vi "integration_code_python.vi"(1 "path de l'image":string, 2 "IDs acceptés":dbl[](array[numeric])) -> (0 "validation":bool)   [LabVIEW 2020]
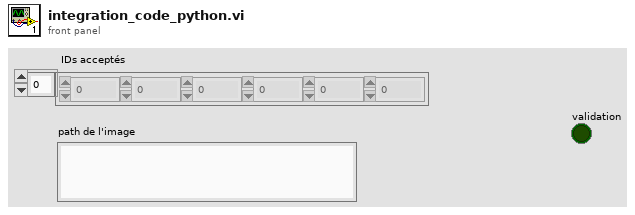
[diagram p1: front panel]
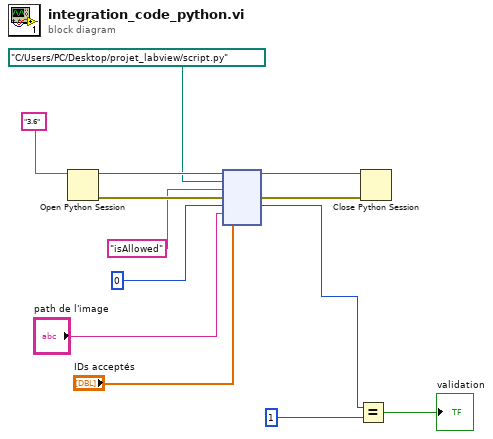
[diagram p0: block diagram]
diagram:
  n1 = Open Python Session(python version="3.6" ("Python version")) -> (session out=w13:refnum<k35>, error out=w12:errorcluster)  [unwired: 2 in]
  n2 = node(w13, path "C:/Users/PC/Desktop/projet_labview/script.py" ("module path"), "isAllowed" ("function name"), w12, 0, "path de l'image", "IDs acceptés") -> (w10:refnum<k35>, w11:errorcluster, w3:i32)  [unwired: 2 in, 2 out]
  n3 = Equal?(x=w3, y=1) -> (x = y?=→"validation":bool)
  n4 = Close Python Session(session in=w10, error in=w11) -> ()  [unwired: 1 out]
